vi "sender_tcp.vi"(11 "Cluster":T1) -> ()   [LabVIEW 2013]
panel:
  in  "Client Closed":string="The client VI closed the connection."
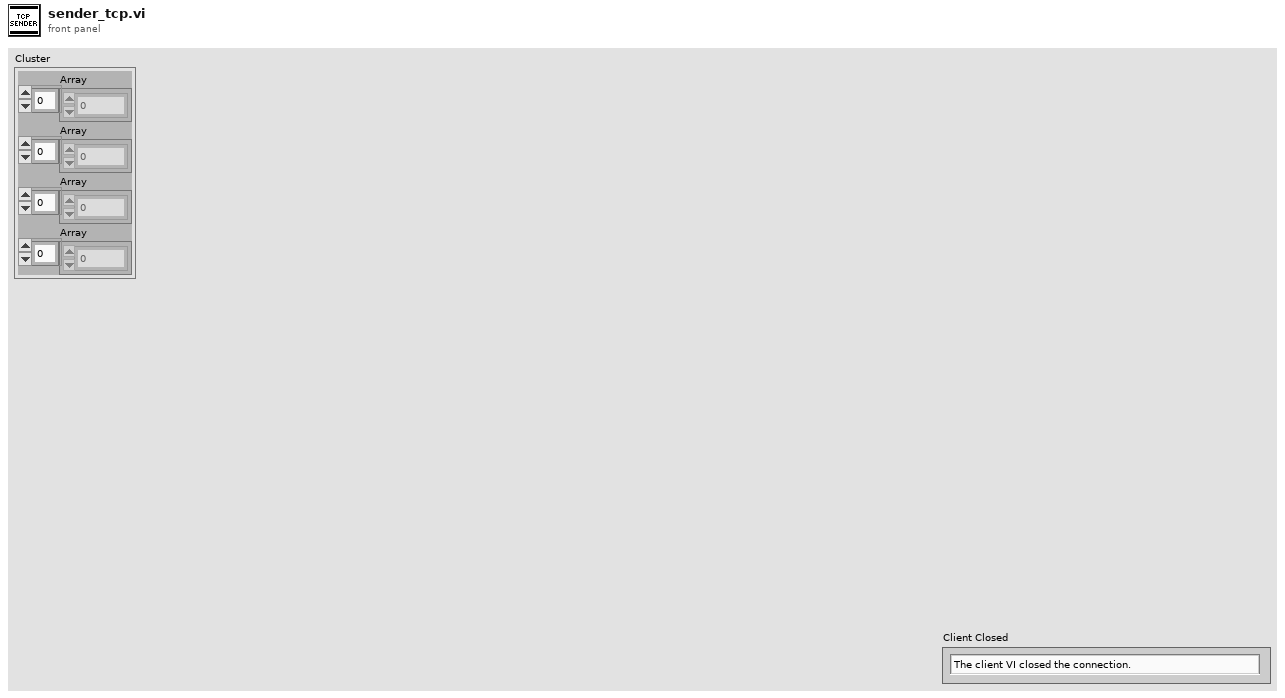
[diagram p1: front panel]
types:
  T1 = cluster{"Array":dbl[], "Array":dbl[], "Array":dbl[], "Array":dbl[]}
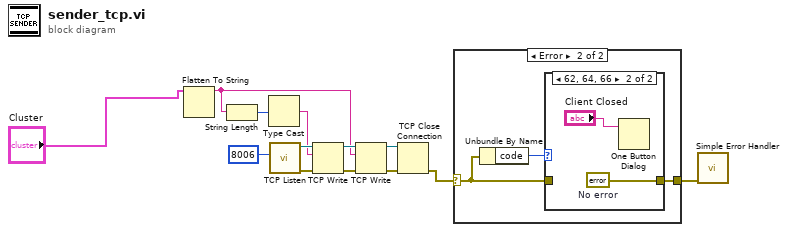
[diagram p0: block diagram]
diagram:
  n1 = Flatten To String(anything="Cluster") -> (data string=w6:string)  [unwired: 3 in, 2 out]
  n2 = String Length(string=w6) -> (length=w8:i32)
  n3 = Type Cast(x=w8) -> (*(type *) &x=w7:string)  [unwired: 1 in]
  n4 = call <vilib>:"TCP Listen.vi"("port"=8006) -> ("error out"=w3:errorcluster, "connection ID"=w11:refnum<k5>)  [unwired: 6 in, 3 out]
  n5 = TCP Write(connection ID=w11, data in=w7, error in (no error)=w3) -> (connection ID out=w10:refnum<k5>, error out=w5:errorcluster)  [unwired: 1 in, 1 out]
  n6 = TCP Write(connection ID=w10, data in=w6, error in (no error)=w5) -> (connection ID out=w9:refnum<k5>, error out=w4:errorcluster)  [unwired: 1 in, 1 out]
  n7 = TCP Close Connection(connection ID=w9, error in (no error)=w4) -> (error out=w1:errorcluster)  [unwired: 1 in, 1 out]
  n8 = case shown="Error" w1 {
    selector: w1 -> [w14 w16]
    tunnel: [w14 w15] -> w2
    frame No Error {
    }
    frame Error {
      n9 = Unbundle By Name(w16) -> ("code"=w17:i32)
      n10 = case shown="62, 64, 66" w17 {
        tunnel: w16 -> [w18 _]
        tunnel: [w18 w20] -> w15
        frame Default {
        }
        frame 62, 64, 66 {
          w20 = errorcluster {"status"=FALSE, "code"=0, "source"=""}  # No error
          n11 = One Button Dialog(message="Client Closed") -> ()  [unwired: 1 in, 1 out]
        }
      }
    }
  }
  n12 = call <vilib>:"Simple Error Handler.vi"("error in (no error)"=w2) -> ()  [unwired: 1 in, 8 out]
